vi "RenameDynamicSignals.vi"(3 "error in":errorcluster, 4 "New Signal Names":string[](array[string])=["SIGNAL_1", "SIGNAL_2", "SIGNAL3"], 5 "Dynamic Data In":dynamicdata(waveform)) -> (0 "error out":errorcluster, 2 "Dynamic Data Out":dynamicdata(waveform))   [LabVIEW 2022 SP3]
doc: "Change the signal names of <B>Dynamic Data In</B> according to the names in the <B>New Signal Names</B> array.\nIf this array contains empty strings or is not long enough, the according signals keep their original names."
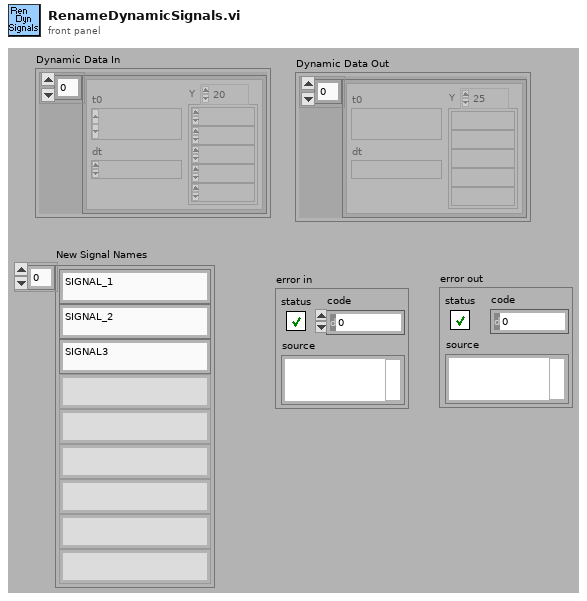
[diagram p1: front panel]
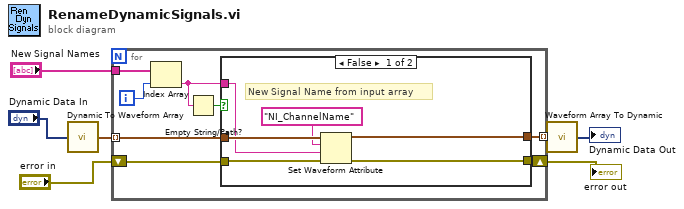
[diagram p0: block diagram]
diagram:
  n1 = call <vilib>:"Dynamic To Waveform Array.vi"("Input"="Dynamic Data In") -> ("Output"=w6:waveform(dbl)[])  [unwired: 4 in]
  n2 = for {
    tunnel: w6 -> [w12] mode=indexing
    tunnel: "New Signal Names" -> [w15]
    shift-right: [w9] -> w3
    shift-left: "error in" -> [w11]
    tunnel: [w8] -> w1 mode=indexing
    i -> [w14]
    n3 = Index Array(array=w15, index=w14) -> (element=w10:string)
    n4 = Empty String/Path?(string/path=w10) -> (empty?=w13:bool)
    n5 = case shown="False" w13 {
      tunnel: w12 -> [w21 w23]
      tunnel: w11 -> [w20 w22]
      tunnel: [w17 w22] -> w9
      tunnel: [w18 w23] -> w8
      tunnel: w10 -> [w19 _]
      frame False {
        # "New Signal Name from input array"
        n6 = Set Waveform Attribute(4:w20, 5:w19, 6:"NI_ChannelName", 7:w21) -> (0:w17:errorcluster, 3:w18:waveform(dbl))  [unwired: 1 out]
      }
      frame True {
        # "No Signal Name in input array.\nUse original Signal Name."
      }
    }
  }
  "error out" <- w3
  n7 = call <vilib>:"Waveform Array To Dynamic.vi"("Input"=w1) -> ("Output"=→"Dynamic Data Out":dynamicdata)  [unwired: 4 in]
